vi "build.vi"(9 "dt":dbl=5e-08 caption="dt (s)" format="%#_6p", 10 "output_settings":T3={"phase_c"=-0.25, "ramp ends"=TRUE, "ramp time"=1e-05, "add func"=FALSE, "f(x)"="-3 * exp(-(x-8E-5)^2/(2 * (1E-6^2)))"} {"ramp time" format="%#_6p"}, 11 "beam settings":T2={"initial velocity"=2000.0, "cell length"=0.025, "electrodes/ cell"=5, "stages"=[{"final vel. (m/s)"=0.0, "distance (m)"=0.05, "hold (s)"=1e-05}, {"final vel. (m/s)"=1250.0, "distance (m)"=0.025, "hold (s)"=0.0}]} {"cell length" format="%#_6p"; "initial velocity" format="%#_6p"; "stages"."hold (s)" format="%#_6p"; "stages"."distance (m)" format="%#_6p"; "stages"."final vel. (m/s)" format="%#_6p"}) -> (0 "num_steps":i32=2650, 1 "corr_wf":dbl[](array[numeric]), 2 "el_wf":dbl[][](array[numeric]), 3 "valid":bool=TRUE, 5 "stats.":T1={"total t"=0.0001325, "total d"=0.125, "max a"=40000000.0} {"total d" format="%#_6p"; "total t" format="%#_6p"})   [LabVIEW 2013, in "wf_tools.lvlib"]
uses:
  wf_tools.lvlib
  stage.ctl
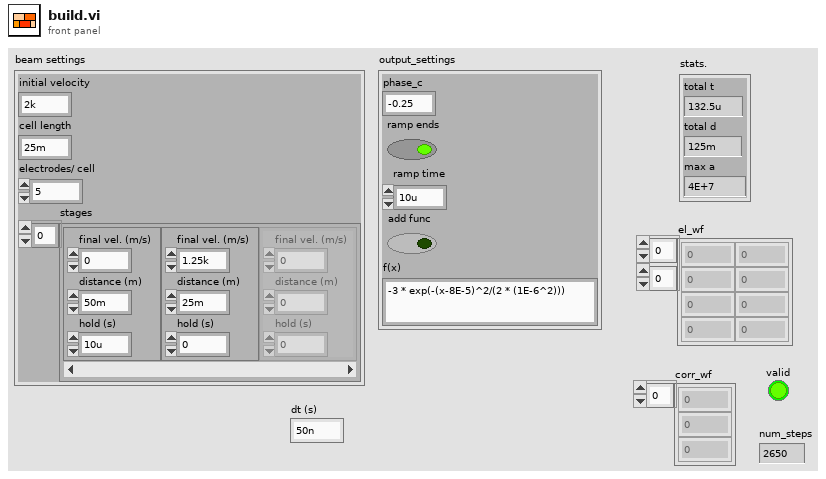
[diagram p1: front panel]
types:
  T1 = cluster{"total t":dbl, "total d":dbl, "max a":dbl}
  T2 = cluster{"initial velocity":dbl, "cell length":dbl, "electrodes/ cell":i32, "stages":cluster{"final vel. (m/s)":dbl, "distance (m)":dbl, "hold (s)":dbl}[]}
  T3 = cluster{"phase_c":dbl, "ramp ends":bool, "ramp time":dbl, "add func":bool, "f(x)":string}
  T4 = cluster{"final vel. (m/s)":dbl, "distance (m)":dbl, "hold (s)":dbl}[]
  T5 = cluster{"total d":dbl, "total t":dbl, "max a":dbl}
  T6 = typedef "wf_tools.lvlib/stage.ctl" = cluster{"v_i (m/s)":dbl, "v_f (m/s)":dbl, "a (m / s^2)":dbl, "d (m)":dbl, "t (s)":dbl}
  T7 = cluster{"time":dbl[], "position":dbl[], "velocity":dbl[]}
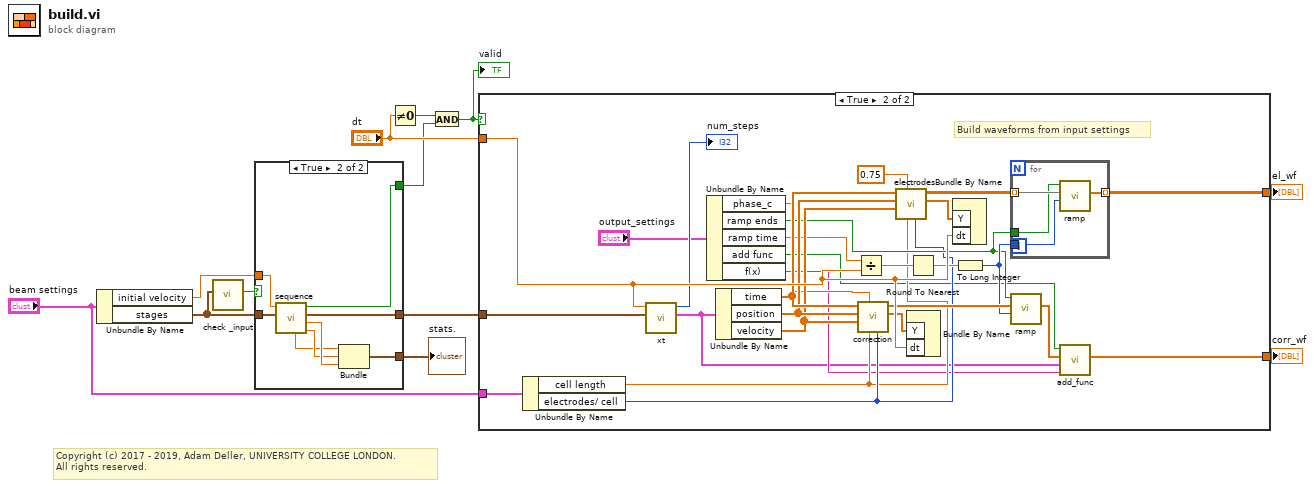
[diagram p0: block diagram]
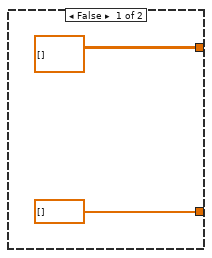
[diagram p2: hidden frame]
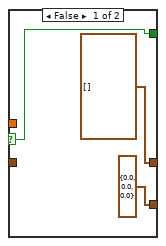
[diagram p3: hidden frame]
diagram:
  # "Copyright (c) 2017 - 2019, Adam Deller, UNIVERSITY COLLEGE LONDON.\nAll rights reserved."
  n1 = Unbundle By Name("beam settings") -> ("initial velocity"=w4:dbl, "stages"=w6:T4)
  n2 = call "check _input.vi"("input"=w6) -> ("valid"=w9:bool)  [unwired: 10 in]
  n3 = case shown="True" w9 {
    selector: w9 -> [w15 _]
    tunnel: w6 -> [_ w23]
    tunnel: [w15 w22] -> w7
    tunnel: [T6[] [] ("stages") w21] -> w11
    tunnel: w4 -> [_ w20]
    tunnel: [T5 {"total d"=0.0, "total t"=0.0, "max a"=0.0} w16] -> w3
    frame False {
    }
    frame True {
      n4 = call "sequence.vi"("input"=w23, "initial vel."=w20) -> ("total t"=w18:dbl, "max a"=w19:dbl, "stages"=w21:T6[], "valid"=w22:bool, "total d"=w17:dbl)  [unwired: 5 in]
      n5 = Bundle("total d"=w17, "total t"=w18, "max a"=w19) -> (w16:T5)  [unwired: 1 in]
    }
  }
  "stats." <- w3
  n6 = Not Equal To 0?(x="dt") -> (x != 0?=w8:bool)
  n7 = And(x=w8, y=w7) -> (x .and. y?=w10:bool)
  "valid" <- w10
  n8 = case shown="True" w10 {
    tunnel: "dt" -> [_ w52]
    tunnel: w11 -> [_ w51]
    tunnel: "beam settings" -> [_ w34]
    tunnel: [dbl[] [] ("wf_out") w29] -> w1
    tunnel: [dbl[][] [] ("wf_out") w28] -> w2
    frame False {
    }
    frame True {
      # "Build waveforms from input settings"
      n9 = Unbundle By Name(w34) -> ("cell length"=w32:dbl, "electrodes/ cell"=w33:i32)
      n10 = call "xt.vi"("stages"=w51, "dt (s)"=w52) -> ("output"=w26:T7, "num_steps"=→"num_steps":i32)  [unwired: 7 in, 1 out]
      n11 = Unbundle By Name("output_settings") -> ("phase_c"=w30:dbl, "ramp ends"=w36:bool, "ramp time"=w35:dbl, "add func"=w31:bool, "f(x)"=w27:string)
      n12 = Unbundle By Name(w26) -> ("time"=w47:dbl[], "position"=w46:dbl[], "velocity"=w45:dbl[])
      n13 = Divide(x=w35, y=w52) -> (x/y=w40:dbl)
      n14 = call "correction.vi"("electrodes/ cell"=w33, "cell length (m)"=w32, "phase / 2 pi"=w30, "velocity"=w45, "position"=w46, "time"=w47) -> ("frequency"=w50:dbl[], "waveform"=w44:dbl[])  [unwired: 4 in]
      n15 = call "electrodes.vi"("electrodes/ cell"=w33, "cell length (m)"=w32, "phase / 2 pi"=0.75, "velocity"=w45, "position"=w46, "time"=w47) -> ("frequency"=w49:dbl[], "waveforms"=w43:dbl[][])  [unwired: 4 in]
      n16 = Bundle By Name("Y"=w50, "dt"=w52) -> ()  [unwired: 1 in, 1 out]
      n17 = Round To Nearest(number=w40) -> (nearest integer value=w39:dbl)
      n18 = Bundle By Name("Y"=w49, "dt"=w52) -> ()  [unwired: 1 in, 1 out]
      n19 = To Long Integer(number=w39) -> (32bit integer=w38:i32)
      n20 = for {
        tunnel: w43 -> [w56] mode=indexing
        tunnel: [w55] -> w28 mode=indexing
        tunnel: w36 -> [w54]
        tunnel: w38 -> [w53]
        n21 = call "ramp.vi"("num_steps"=w53, "wf_in"=w56, "apply"=w54) -> ("wf_out"=w55:dbl[])  [unwired: 8 in]
      }
      n22 = call "ramp.vi"("num_steps"=w38, "wf_in"=w44, "apply"=w36) -> ("wf_out"=w41:dbl[])  [unwired: 8 in]
      n23 = call "add_func.vi"("f(x, t)"=w27, "output"=w26, "wf_in"=w41, "apply"=w31) -> ("wf_out"=w29:dbl[])  [unwired: 6 in, 1 out]
    }
  }
  "corr_wf" <- w1
  "el_wf" <- w2
